vi "getEndScriptEvent.vi"(8 "error in (no error)":errorcluster, 11 "RampEvent.lvclass in":refnum<class "RampEvent.lvclass">) -> (0 "error out":errorcluster, 2 "ScriptEvent.lvclass":refnum<class "ScriptEvent.lvclass">, 3 "RampEvent.lvclass out":refnum<class "RampEvent.lvclass">)   [LabVIEW 2011, in "Tools.lvlib" / "Scripting.lvlib" / "RampEvent.lvclass"]
uses:
  RampEvent.lvclass
  ScriptEvent.lvclass
  RampEvent.lvclass/RampEvent.ctl
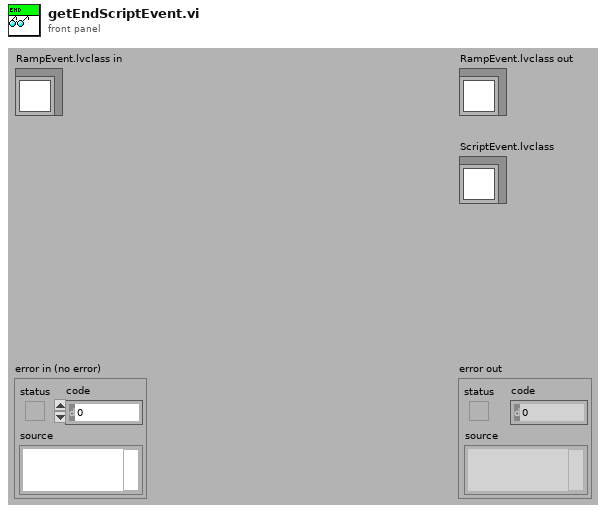
[diagram p1: front panel]
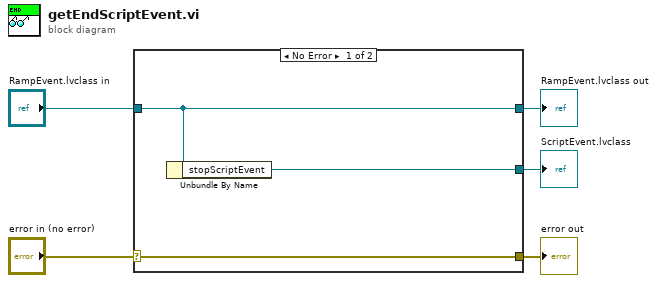
[diagram p0: block diagram]
diagram:
  n1 = case shown="No Error" "error in (no error)" {
    selector: "error in (no error)" -> [w8 w9]
    tunnel: [w8 w9] -> w4
    tunnel: [w7 w10] -> w2
    tunnel: "RampEvent.lvclass in" -> [w7 w10]
    tunnel: [w6 _] -> w1
    frame No Error {
      n2 = Unbundle By Name(w7) -> ("stopScriptEvent"=w6:refnum<class "ScriptEvent.lvclass">)
    }
    frame Error {
    }
  }
  "error out" <- w4
  "RampEvent.lvclass out" <- w2
  "ScriptEvent.lvclass" <- w1
